vi "Configuration.vi"(6 "Return Data":refnum<user-event>, 8 "error in (no error)":errorcluster, 9 "Exit Running Config":refnum<user-event>, 10 "Panel in":refnum<class "Panel.lvclass">, 11 "List Data Type in":refnum<class "List Data Type.lvclass">) -> (0 "error out":errorcluster, 3 "List Data Type out":refnum<class "List Data Type.lvclass">)   [LabVIEW 2018, in "List Data Type.lvclass"]
uses:
  List Data Type.lvclass
  D:/Code/QControls Extended/DataGrid/DataGrid Configuration/Data Type Classes/Generic/Generic Data Type.lvclass
  <vilib>/MGI/Panel Manager/Panel/Panel/Panel.lvclass
  Generic/Generic Data Type.lvclass
  List Data Type.lvclass/List Data Type.ctl
  Generic/Generic Data Type.lvclass/Generic Data Type.ctl
  Generic/Write Column Header.vi
  Generic/Read Column Header.vi
panel:
  in  "Auto Sort List":bool
  in  "Column Header":string
  in  "Allow Undefined Strings":bool
  in  "Add NULL Value":bool
  in  "Default Value":string(combo)
  in  "Drop-down List Options":string[](array[string])
  # "Drop-Down List Column"
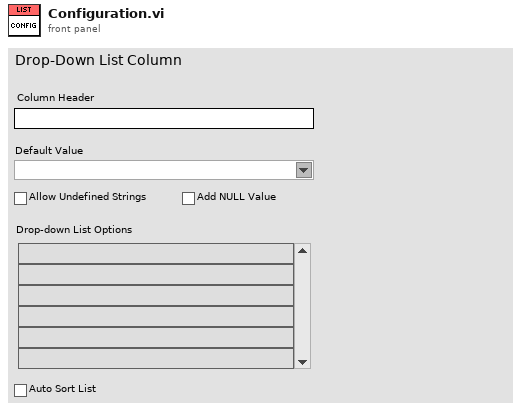
[diagram p1: front panel]
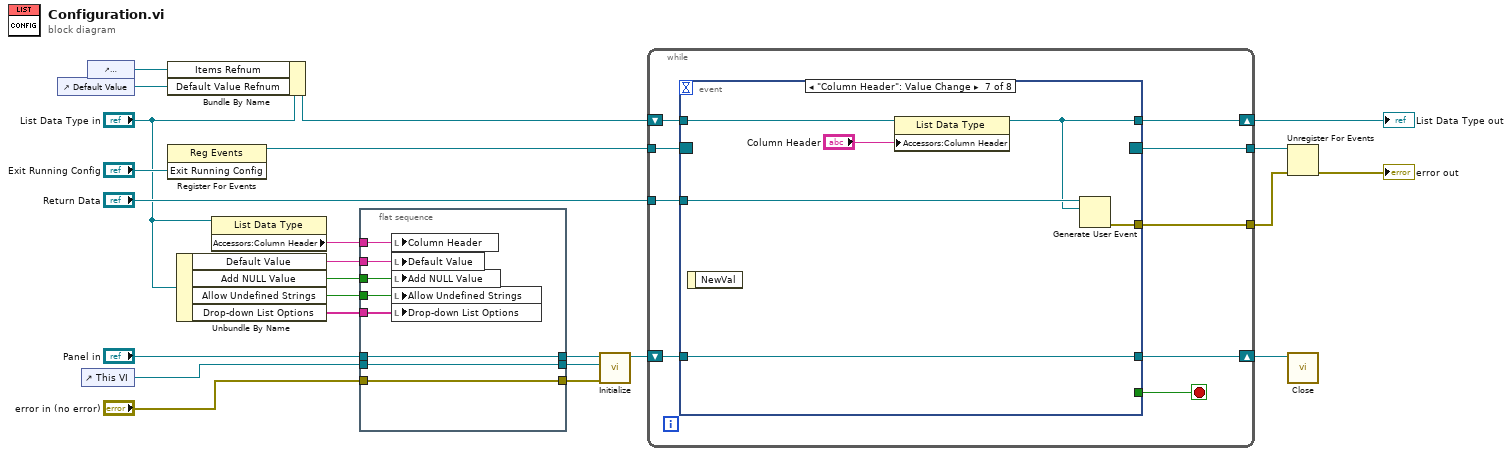
[diagram p0: block diagram]
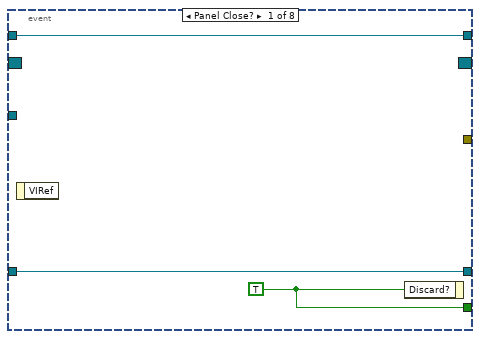
[diagram p2: hidden frame]
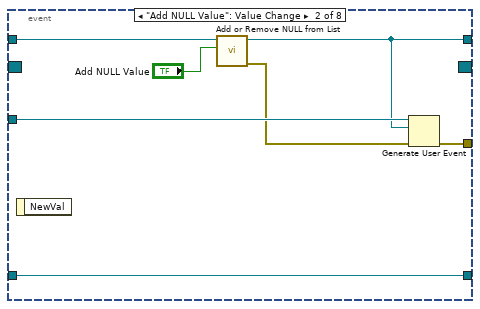
[diagram p3: hidden frame]
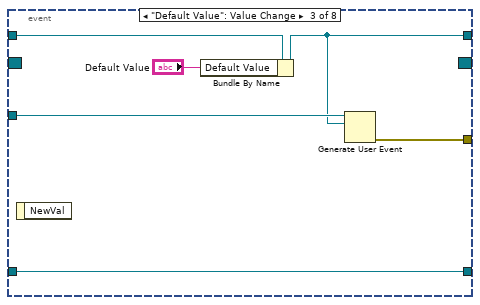
[diagram p4: hidden frame]
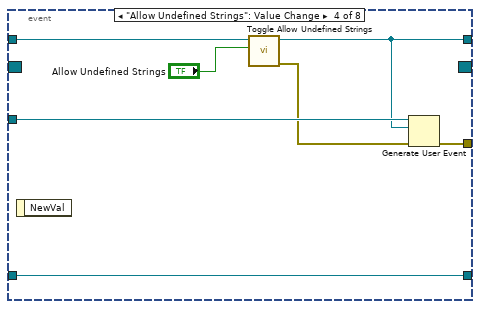
[diagram p5: hidden frame]
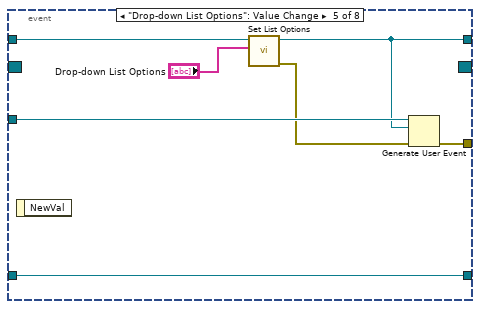
[diagram p6: hidden frame]
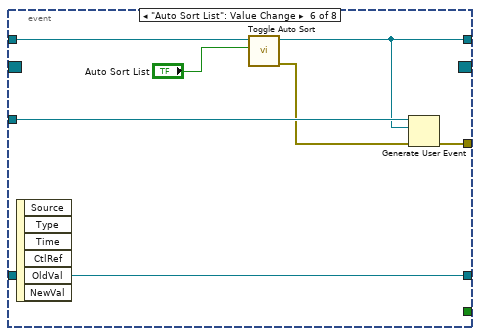
[diagram p7: hidden frame]
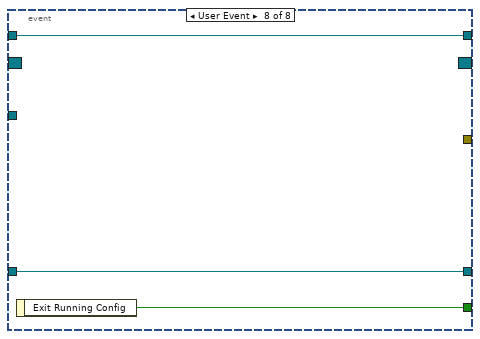
[diagram p8: hidden frame]
diagram:
  n1 = control-ref of="Default Value"() -> (w4:refnum<vi>)
  n2 = control-ref of="This VI"() -> (w20:refnum<vi>)
  n3 = control-ref of="Drop-down List Options"() -> (w1:refnum<vi>)
  n4 = Bundle By Name(cluster="List Data Type in", "Items Refnum"=w1, "Default Value Refnum"=w4) -> (w2:refnum<class "List Data Type.lvclass">)
  n5 = register-events("Exit Running Config") -> (reference out=w14:refnum<event-registration>)  [unwired: 2 in, 1 out]
  n6 = Unbundle By Name("List Data Type in") -> ("Default Value"=w23:string, "Add NULL Value"=w17:bool, "Allow Undefined Strings"=w6:bool, "Drop-down List Options"=w5:string[])
  n7 = property class="List Data Type"(reference="List Data Type in") -> ("Accessors:Column Header"=w24:string)  [unwired: 1 in, 2 out]
  n8 = flat-sequence {
    tunnel: w17 -> [w32]
    tunnel: "Panel in" -> [w31]
    tunnel: [w31] -> w18
    tunnel: [w30] -> w19
    tunnel: w20 -> [w30]
    tunnel: "error in (no error)" -> [w29]
    tunnel: [w29] -> w22
    tunnel: w23 -> [w28]
    tunnel: w24 -> [w27]
    tunnel: w6 -> [w26]
    tunnel: w5 -> [w25]
    frame #0 {
      n9 = local write "Column Header"(w27) -> ()
      n10 = local write "Default Value"(w28) -> ()
      n11 = local write "Add NULL Value"(w32) -> ()
      n12 = local write "Allow Undefined Strings"(w26) -> ()
      n13 = local write "Drop-down List Options"(w25) -> ()
    }
  }
  n14 = call <vilib>:"Initialize.vi"("error in (no error)"=w22, "VI Refnum"=w19, "Panel In"=w18) -> ("Panel Out"=w16:refnum<class "Panel.lvclass">)  [unwired: 6 in, 2 out]
  n15 = while {
    shift-right: [w35] -> w12
    shift-left: w2 -> [w41]
    shift-right: [w37] -> w15
    shift-left: w16 -> [w38]
    tunnel: w14 -> [w39]
    tunnel: [w36] -> w13
    tunnel: "Return Data" -> [w34]
    tunnel: [w33] -> w21
    stop <- w40 stop-if-true
    n16 = event shown="[6] \"Column Header\": Value Change" {
      selector: w39 -> [_ _ _ _ _ _ _ _]
      dyn-events: [_ _ _ _ _ _ _ _] -> w36
      timeout: _ -> [_ _ _ _ _ _ _ _]
      tunnel: w41 -> [w44 w47 w56 w61 w68 w75 w81 w87]
      tunnel: [w44 w48 w54 w60 w67 w74 w80 w87] -> w35
      tunnel: [w43 _ _ _ _ _ _ w86] -> w40
      tunnel: w38 -> [w42 w51 w57 w64 w71 w78 w84 w85]
      tunnel: [w42 w51 w57 w64 w71 w78 w84 w85] -> w37
      tunnel: w34 -> [_ w50 w55 w63 w70 w77 w83 _]
      tunnel: [_ w49 w53 w62 w69 w76 w82 _] -> w33
      event Panel Close? {
        w43 = TRUE
        n17 = event-data() -> ()  [unwired: 1 in, 1 out]
        n18 = event-data("Discard?"=w43) -> ()  [unwired: 1 in, 1 out]
      }
      event "Add NULL Value": Value Change {
        n19 = event-data() -> ()  [unwired: 1 in, 1 out]
        n20 = call "Add or Remove NULL from List.vi"("Add NULL Value"="Add NULL Value", "List Data Type in"=w47) -> ("error out"=w45:errorcluster, "List Data Type out"=w48:refnum<class "List Data Type.lvclass">)  [unwired: 8 in]
        n21 = Generate User Event(user event=w50, event data cluster=w48, error in=w45) -> (error out=w49:errorcluster)  [unwired: 1 in, 1 out]
      }
      event "Default Value": Value Change {
        n22 = event-data() -> ()  [unwired: 1 in, 1 out]
        n23 = Bundle By Name(cluster=w56, "Default Value"="Default Value") -> (w54:refnum<class "List Data Type.lvclass">)
        n24 = Generate User Event(user event=w55, event data cluster=w54) -> (error out=w53:errorcluster)  [unwired: 2 in, 1 out]
      }
      event "Allow Undefined Strings": Value Change {
        n25 = event-data() -> ()  [unwired: 1 in, 1 out]
        n26 = call "Toggle Allow Undefined Strings.vi"("Allow Undefined Strings"="Allow Undefined Strings", "List Data Type in"=w61) -> ("error out"=w58:errorcluster, "List Data Type out"=w60:refnum<class "List Data Type.lvclass">)  [unwired: 8 in]
        n27 = Generate User Event(user event=w63, event data cluster=w60, error in=w58) -> (error out=w62:errorcluster)  [unwired: 1 in, 1 out]
      }
      event "Drop-down List Options": Value Change {
        n28 = event-data() -> ()  [unwired: 1 in, 1 out]
        n29 = call "Set List Options.vi"("Drop-down List Options"="Drop-down List Options", "List Data Type in"=w68) -> ("error out"=w65:errorcluster, "List Data Type out"=w67:refnum<class "List Data Type.lvclass">)  [unwired: 8 in]
        n30 = Generate User Event(user event=w70, event data cluster=w67, error in=w65) -> (error out=w69:errorcluster)  [unwired: 1 in, 1 out]
      }
      event "Auto Sort List": Value Change {
        n31 = event-data() -> ()  [unwired: 1 in, 6 out]
        n32 = call "Toggle Auto Sort.vi"("Auto Sort"="Auto Sort List", "List Data Type in"=w75) -> ("error out"=w73:errorcluster, "List Data Type out"=w74:refnum<class "List Data Type.lvclass">)  [unwired: 8 in]
        n33 = Generate User Event(user event=w77, event data cluster=w74, error in=w73) -> (error out=w76:errorcluster)  [unwired: 1 in, 1 out]
      }
      event "Column Header": Value Change {
        n34 = event-data() -> ()  [unwired: 1 in, 1 out]
        n35 = property class="List Data Type"(reference=w81, "Accessors:Column Header"="Column Header") -> (reference out=w80:refnum<class "List Data Type.lvclass">)  [unwired: 1 in, 1 out]
        n36 = Generate User Event(user event=w83, event data cluster=w80) -> (error out=w82:errorcluster)  [unwired: 2 in, 1 out]
      }
      event User Event {
        n37 = event-data() -> ("Exit Running Config"=w86:bool)  [unwired: 1 in]
      }
    }
  }
  "List Data Type out" <- w12
  n38 = Unregister For Events(event registration refnum=w13, error in=w21) -> (error out=→"error out":errorcluster)
  n39 = call-dynamic "Close.vi"("Panel In"=w15) -> ()  [unwired: 10 in, 1 out]
